vi "MH_SetInputChannelEnable.vi"(8 "error in (no error)":errorcluster, 9 "enable":bool, 10 "channel":i32, 11 "devidx":i32) -> (0 "error out":errorcluster, 3 "return type":i32)   [LabVIEW 2019]
uses:
  <userlib>/MultiHarp150/MH_DllPath_global.vi
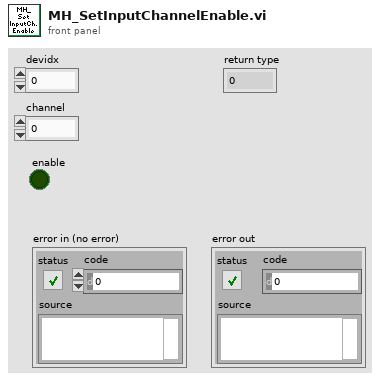
[diagram p1: front panel]
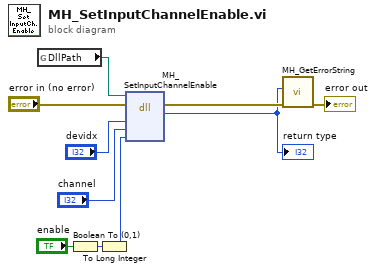
[diagram p0: block diagram]
diagram:
  n1 = global read "MH_DllPath_global.vi" "DllPath"() -> (w9:path)
  n2 = Boolean To (0,1)(Boolean="enable") -> (0, 1=w2:i16)
  n3 = To Long Integer(number=w2) -> (32bit integer=w1:i32)
  n4 = dll-call lib="MHLib64.dll" fn="MH_SetInputChannelEnable"(path in=w9, error in="error in (no error)", "devidx"="devidx", "channel"="channel", "enable"=w1) -> (error out=w7:errorcluster, "return type"=w6:i32)  [unwired: 4 in, 1 out]
  "return type" <- w6
  n5 = call <userlib>:"MH_GetErrorString.vi"("error in (no error)"=w7, "code"=w6) -> ("error out"=→"error out":errorcluster)  [unwired: 7 in, 2 out]
